vi "test1ad.vi"() -> ()   [LabVIEW 2016]
uses:
  <vilib>/Utility/miscctls.llb/LVComboBoxStrsAndValuesArrayTypeDef.ctl
  <vilib>/addons/database/Connection.llb/DB Tools Open Connec (String).vi
  <vilib>/addons/database/Connection.llb/Conn Execute.vi
  <vilib>/addons/database/Recordset.llb/Rec Fetch Recordset Data (R).vi
  <vilib>/addons/database/Recordset.llb/Rec Destroy - Connection.vi
  <vilib>/addons/database/NI_Database_API.lvlib
panel:
  out "Array 3":string[](array[string])
  out "Array 2":string[](array[string])
  out "Array":string[][](array[string])
  in  "Combo Box":string(combo)
  out "error out":errorcluster
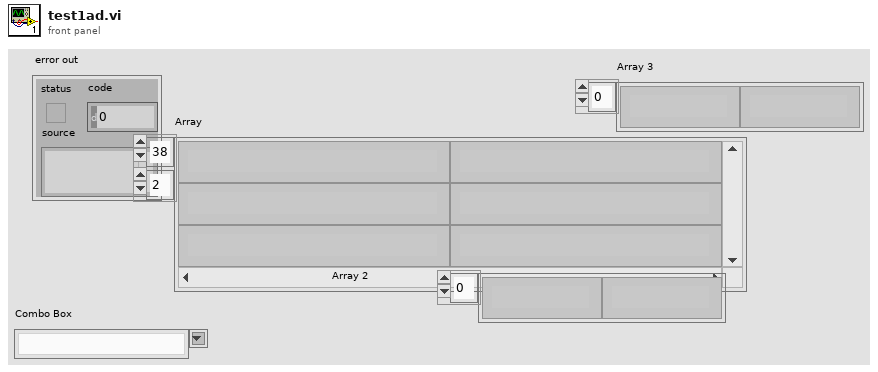
[diagram p1: front panel]
types:
  T1 = typedef "LVComboBoxStrsAndValuesArrayTypeDef.ctl" = cluster{"String":string, "Value":string}[]
  T2 = typedef "NI_Database_API.lvlib/Conn ObjectReference.ctl" = refnum<k1>
  T3 = typedef "NI_Database_API.lvlib/Rec ObjectReference.ctl" = refnum<k1>
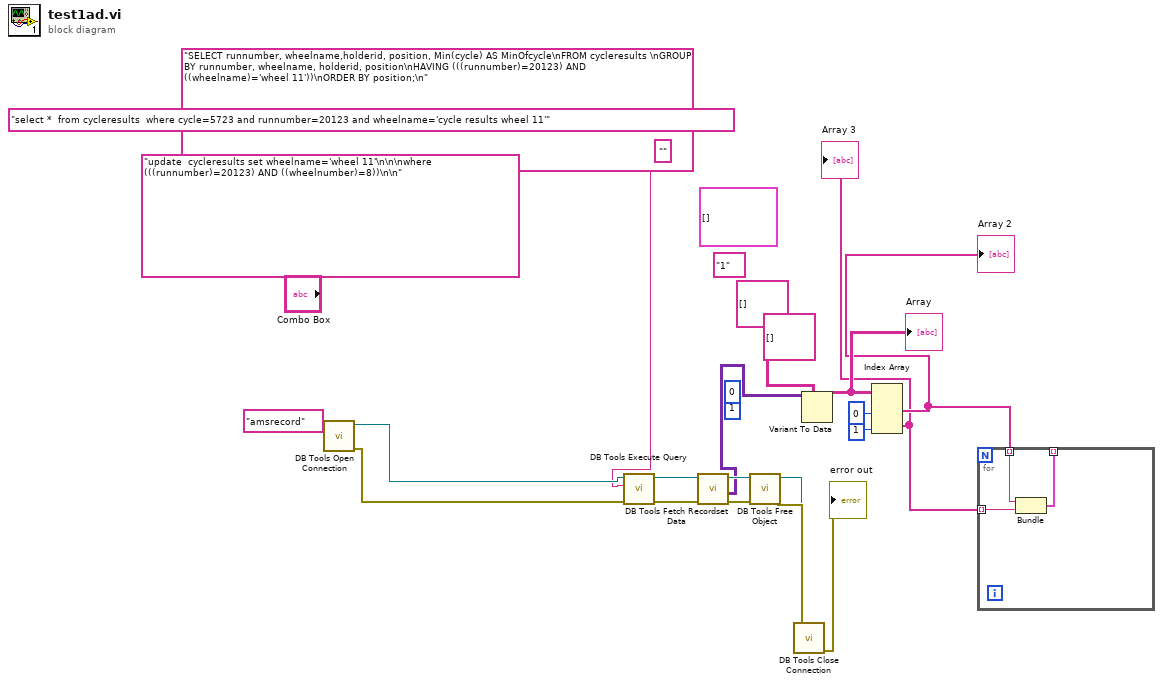
[diagram p0: block diagram]
diagram:
  (unwired) "select *  from cycleresults  where cycle=5723 and runnumber=20123 and wheelname='cycle results wheel 11'" ("SQL query")
  (unwired) string[][] [] ("Strings []")
  (unwired) T1 [] ("Strings And Values []")
  (unwired) "" ("SQL query")
  (unwired) 1 ("disabled index (col)")
  (unwired) "1" ("wheelnumber")
  (unwired) 0 ("disabled index (col)")
  (unwired) "update  cycleresults set wheelname='wheel 11'\n\n\nwhere  (((runnumber)=20123) AND ((wheelnumber)=8))\n\n" ("SQL query")
  n1 = call-poly <vilib>:"DB Tools Open Connection.vi"("connection information"="amsrecord") -> ("error out"=w4:errorcluster, "connection reference"=w13:T2)  [unwired: 7 in]
  n2 = call-poly <vilib>:"DB Tools Execute Query.vi"("error in (no error)"=w4, "SQL query"="SELECT runnumber, wheelname,holderid, position, Min(cycle) AS MinOfcycle\nFROM cycleresults \nGROUP BY runnumber, wheelname, holderid, position\nHAVING (((runnumber)=20123) AND ((wheelname)='wheel 11'))\nORDER BY position;\n", "connection reference"=w13) -> ("error out"=w16:errorcluster, "recordset reference"=w14:T3)  [unwired: 5 in]
  n3 = call-poly <vilib>:"DB Tools Fetch Recordset Data.vi"("error in (no error)"=w16, "recordset reference"=w14) -> ("error out"=w17:errorcluster, "recordset data"=w6:variant[][], "recordset reference out"=w15:T3)  [unwired: 3 in]
  n4 = call-poly <vilib>:"DB Tools Free Object.vi"("error in (no error)"=w17, "recordset reference"=w15) -> ("error out"=w12:errorcluster, "connection reference"=w11:T2)  [unwired: 8 in]
  n5 = call <vilib>:"DB Tools Close Connection.vi"("error in (no error)"=w12, "connection reference"=w11) -> ("error out"=→"error out":errorcluster)  [unwired: 5 in]
  n6 = Variant To Data(type=string[][] [] ("Strings []"), Variant=w6) -> (data=w5:string[][])  [unwired: 1 in, 1 out]
  "Array" <- w5
  n7 = Index Array(array=w5, index (col) #1=0 ("disabled index (col)"), index (col) #2=1 ("index (col)")) -> (element #1=w3:string[], element #2=w2:string[])  [unwired: 2 in]
  "Array 2" <- w3
  "Array 3" <- w2
  n8 = for {
    tunnel: w3 -> [w21] mode=indexing
    tunnel: w2 -> [w20] mode=indexing
    tunnel: [w19] -> _ mode=indexing
    n9 = Bundle(w21, w20) -> (w19:cluster{string, string})  [unwired: 1 in]
  }
